vi "set Front Panel State.vi"(8 "error in (no error)":errorcluster, 10 "Front Panel State":T1=enum."Standard", 11 "Actor in":refnum<class "Actor.lvclass">) -> (0 "error out":errorcluster, 3 "Actor out":refnum<class "Actor.lvclass">)   [LabVIEW 2015, in "Actor.lvclass"]
uses:
  Actor.lvclass
  Front Panel State.ctl
  Actor.lvclass/Actor.ctl
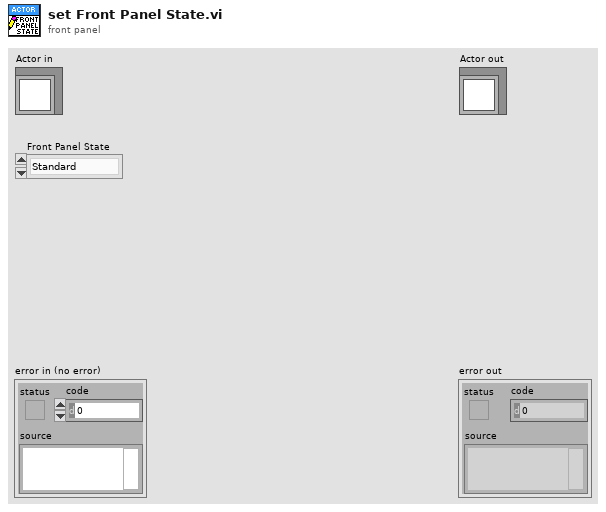
[diagram p1: front panel]
types:
  T1 = typedef "Actor.lvclass/Front Panel State.ctl" = enum32{"Invalid", "Standard", "Closed", "Hidden", "Minimized", "Maximized"}
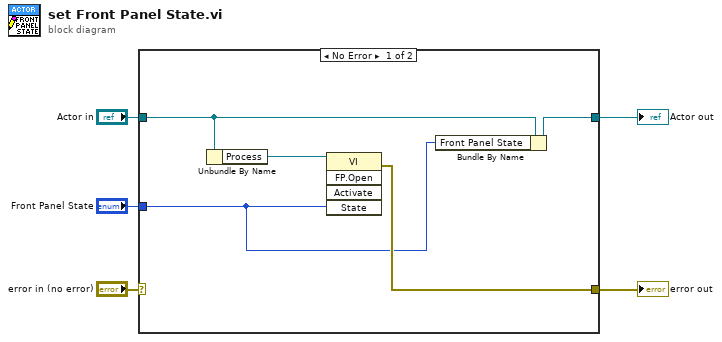
[diagram p0: block diagram]
diagram:
  n1 = case shown="No Error" "error in (no error)" {
    selector: "error in (no error)" -> [_ w11]
    tunnel: [w8 w11] -> w4
    tunnel: [w10 w12] -> w2
    tunnel: "Actor in" -> [w9 w12]
    tunnel: "Front Panel State" -> [w7 _]
    frame No Error {
      n2 = Unbundle By Name(w9) -> ("Process"=w6:refnum<vi>)
      n3 = invoke class="VI" method="FP.Open"(reference=w6, "State"=w7) -> (error out=w8:errorcluster)  [unwired: 3 in, 4 out]
      n4 = Bundle By Name(cluster=w9, "Front Panel State"=w7) -> (w10:refnum<class "Actor.lvclass">)
    }
    frame Error {
    }
  }
  "error out" <- w4
  "Actor out" <- w2
